vi "Servo berekening.vi"(9 "freq [Hz]":dbl, 10 "null offset":bool, 11 "position [%FS] in":dbl) -> (1 "Duty Cycle [%]":dbl, 2 "Puls Width [ms]":dbl, 3 "position [%FS] out":dbl, 4 "Duty Cycle":dbl)   [LabVIEW 2014]
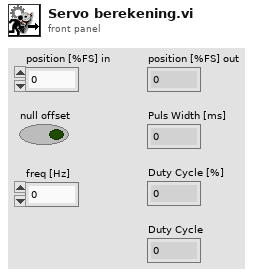
[diagram p1: front panel]
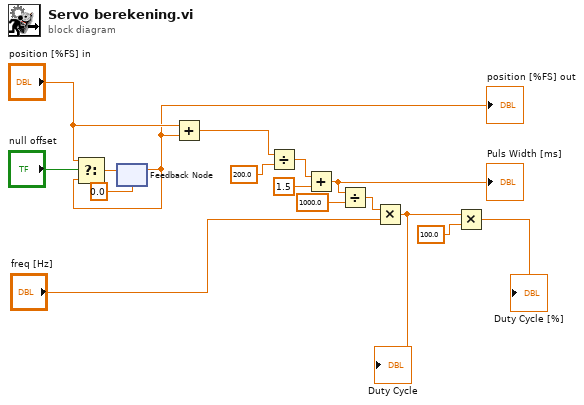
[diagram p0: block diagram]
diagram:
  n1 = feedback #1(0.0 ("position [%FS]")) -> (w10:dbl)
  "position [%FS] out" <- w10
  n2 = Select(t="position [%FS] in", s="null offset", f=w10) -> (s? t:f=w8:dbl)
  n3 = feedback-in #1(w8) -> ()
  n4 = Add(x="position [%FS] in", y=w10) -> (x+y=w9:dbl)
  n5 = Divide(x=w9, y=200.0) -> (x/y=w2:dbl)
  n6 = Add(x=w2, y=1.5) -> (x+y=w4:dbl)
  "Puls Width [ms]" <- w4
  n7 = Divide(x=w4, y=1000.0) -> (x/y=w12:dbl)
  n8 = Multiply(x=w12, y="freq [Hz]") -> (x*y=w15:dbl)
  "Duty Cycle" <- w15
  n9 = Multiply(x=w15, y=100.0) -> (x*y=→"Duty Cycle [%]":dbl)
